vi "encodeMapHeader.vi"(3 "Number of Elements":u32) -> (1 "map header":u8[](array[numeric]) format="%.0x")   [LabVIEW 2015, in "MsgPack.lvlib"]
uses:
  MsgPack.lvlib
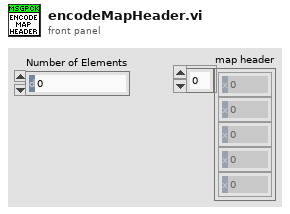
[diagram p1: front panel]
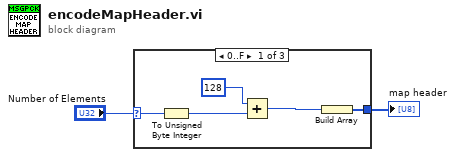
[diagram p0: block diagram]
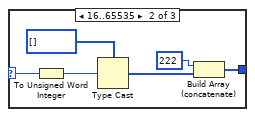
[diagram p2: hidden frame]
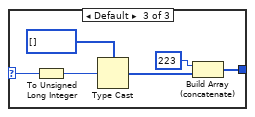
[diagram p3: hidden frame]
diagram:
  n1 = case shown="0..F" "Number of Elements" {
    selector: "Number of Elements" -> [w5 w13 w14]
    tunnel: [w3 w8 w16] -> w2
    frame 0..15 {
      n2 = To Unsigned Byte Integer(number=w5) -> (unsigned 8bit integer=w7:u8)
      n3 = Add(x=u8 128, y=w7) -> (x+y=w4:u8)
      n4 = Build Array(w4) -> (w3:u8[])
    }
    frame 16..65535 {
      n5 = To Unsigned Word Integer(number=w13) -> (unsigned 16bit integer=w11:u16)
      n6 = Type Cast(type=u8[] [], x=w11) -> (*(type *) &x=w9:u8[])
      n7 = Build Array (concatenate)(u8 222 ("x"), w9) -> (w8:u8[])
    }
    frame Default {
      n8 = To Unsigned Long Integer(number=w14) -> (unsigned 32bit integer=w15:u32)
      n9 = Type Cast(type=u8[] [], x=w15) -> (*(type *) &x=w19:u8[])
      n10 = Build Array (concatenate)(u8 223 ("x"), w19) -> (w16:u8[])
    }
  }
  "map header" <- w2
